vi "ExSpectGetSlitInfoMult.vi"() -> ()   [LabVIEW 2010]
panel:
  out "Speed 2":dbl format="%.2f"
  out "Position 2":dbl format="%.2f"
  in  "Slit Number 2":i16=1 min=1 max=4 step=1
  out "Speed":dbl format="%.2f"
  out "Position":dbl format="%.2f"
  in  "Slit Number 1":i16=1 min=1 max=4 step=1
  out "error out":errorcluster
  in  "error in (no error)":errorcluster
  # "ExSpectGetSlitInfo.vi\n(Normal Spectrograph via USB/COM port)\nThis VI will read the current position and speed of the selected slit."
  # "SPECTROMETER 2"
  # "SPECTROMETER 1"
  # "um"
  # "um"
  # "1 = Front Entrance\n 2 = Side Entrance\n 3 = Front Exit\n 4 = Side Exit"
  # "1 = Front Entrance\n 2 = Side Entrance\n 3 = Front Exit\n 4 = Side Exit"
  # "NOTES:\nA properly configured spectometer .ini must be present in the LabVIEW folder for spectrograph operation.\n\nConsult the Toolkit documentation for more information on how to configure this file."
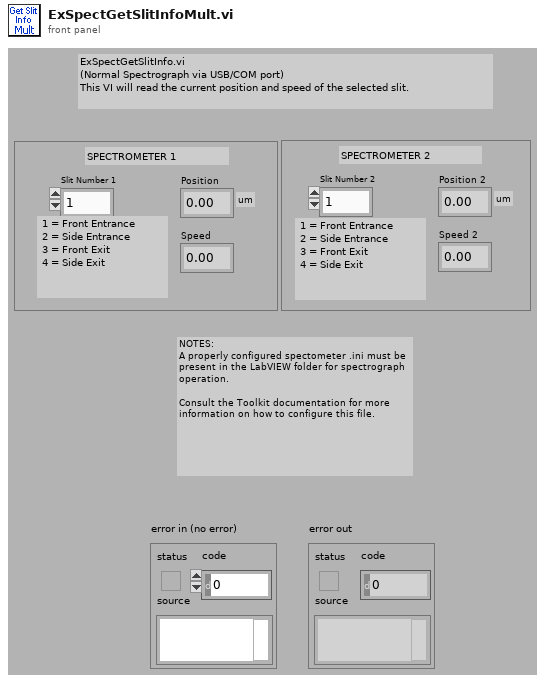
[diagram p1: front panel]
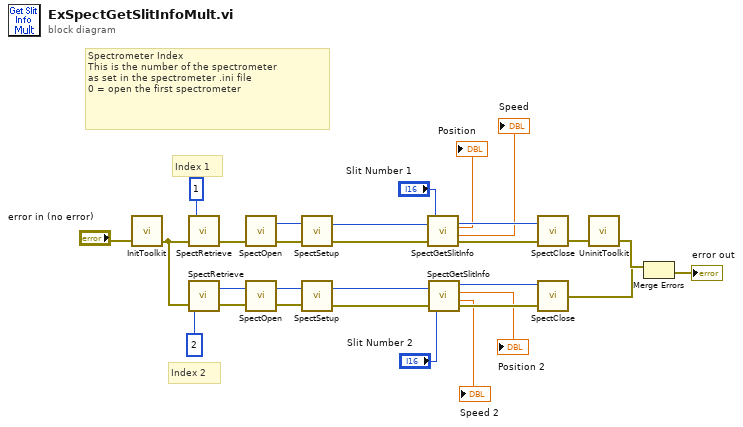
[diagram p0: block diagram]
diagram:
  # "Index 2"
  # "Index 1"
  # "Spectrometer Index\nThis is the number of the spectrometer\nas set in the spectrometer .ini file\n0 = open the first spectrometer"
  n1 = call <userlib>:"InitToolkit.vi"("error in"="error in (no error)") -> ("error out"=w4:errorcluster)
  n2 = call <userlib>:"SpectRetrieve.vi"("error in"=w4, "Index"=1) -> ("error out"=w6:errorcluster)  [unwired: 1 out]
  n3 = call <userlib>:"SpectRetrieve.vi"("error in"=w4, "Index"=2) -> ("error out"=w3:errorcluster, "Device ID"=w1:u32)
  n4 = call <userlib>:"SpectOpen.vi"("error in"=w6) -> ("error out"=w28:errorcluster, "Spectrometer Handle"=w24:u32)  [unwired: 2 in]
  n5 = call <userlib>:"SpectOpen.vi"("error in"=w3, "Spectrometer ID"=w1) -> ("error out"=w18:errorcluster, "Spectrometer Handle"=w12:u32)  [unwired: 1 in]
  n6 = call <userlib>:"SpectSetup.vi"("error in"=w28, "Spectrometer Handle"=w24) -> ("error out"=w27:errorcluster, "Spectrometer Handle"=w23:u32)
  n7 = call <userlib>:"SpectSetup.vi"("error in"=w18, "Spectrometer Handle"=w12) -> ("error out"=w17:errorcluster, "Spectrometer Handle"=w11:u32)
  n8 = call <userlib>:"SpectGetSlitInfo.vi"("Spectrometer Handle"=w23, "Slit"="Slit Number 1", "error in"=w27) -> ("Spectrometer Handle"=w22:u32, "Position"=→"Position":dbl, "Speed"=→"Speed":dbl, "error out"=w26:errorcluster)
  n9 = call <userlib>:"SpectGetSlitInfo.vi"("Spectrometer Handle"=w11, "Slit"="Slit Number 2", "error in"=w17) -> ("Spectrometer Handle"=w10:u32, "Position"=→"Position 2":dbl, "Speed"=→"Speed 2":dbl, "error out"=w16:errorcluster)
  n10 = call <userlib>:"SpectClose.vi"("error in"=w26, "Spectrometer Handle"=w22) -> ("error out"=w25:errorcluster)
  n11 = call <userlib>:"SpectClose.vi"("error in"=w16, "Spectrometer Handle"=w10) -> ("error out"=w14:errorcluster)
  n12 = call <userlib>:"UninitToolkit.vi"("error in"=w25) -> ("error out"=w15:errorcluster)
  n13 = Merge Errors(w15, w14) -> (→"error out":errorcluster)
